vi "Write PID Gains.vi"(0 "VISA Session In":refnum<visa-resource-name>="Alicat", 2 "PID Gain Settings":T1 {"P Gain" min=0 max=65535 step=1; "D Gain" min=0 max=65535 step=1; "I Gain" min=0 max=65535 step=1}, 3 "error in":errorcluster, 4 "Unit ID (A)":string="A") -> (7 "VISA Session Out":refnum<visa-resource-name>, 10 "error out":errorcluster)   [LabVIEW 2016]
doc: "Writes the P, I, and D gains to an Alicat controller."
panel:
  # "Only writes values for \nP, D, & I gains. For other\nvalve tuning options, use \n\"Write PID Settings.vi\""
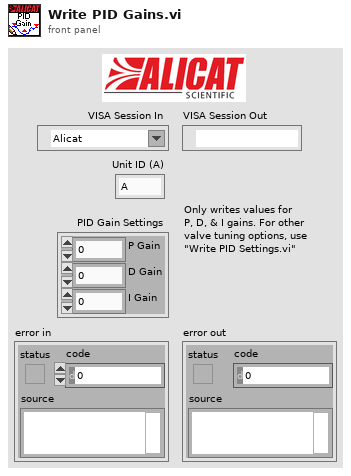
[diagram p1: front panel]
types:
  T1 = cluster{"P Gain":i32, "D Gain":i32, "I Gain":i32}
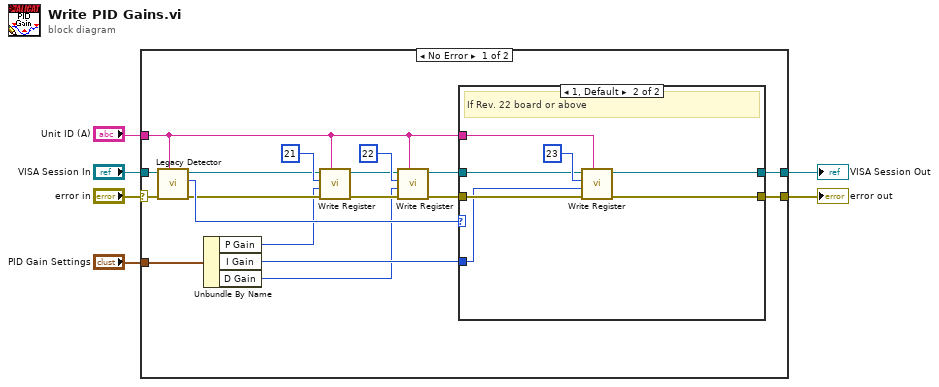
[diagram p0: block diagram]
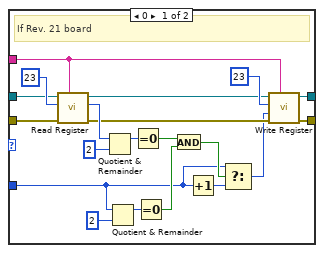
[diagram p2: hidden frame]
diagram:
  n1 = case shown="No Error" "error in" {
    selector: "error in" -> [w23 w52]
    tunnel: [w8 w52] -> w6
    tunnel: [w9 w53] -> w5
    tunnel: "VISA Session In" -> [w24 w53]
    tunnel: "Unit ID (A)" -> [w7 _]
    tunnel: "PID Gain Settings" -> [w22 _]
    frame No Error {
      n2 = call "Legacy Detector.vi"("Unit ID (A)"=w7, "error in"=w23, "VISA Session In"=w24) -> ("error out"=w17:errorcluster, "Legacy Status"=w21:u8, "VISA Session Out"=w16:refnum<visa-resource-name>)  [unwired: 6 in]
      n3 = Unbundle By Name(w22) -> ("P Gain"=w11:i32, "I Gain"=w20:i32, "D Gain"=w10:i32)
      n4 = call "Write Register.vi"("Unit ID (A)"=w7, "error in"=w17, "Register Value"=w11, "Register address"=u16 21, "VISA Session In"=w16) -> ("error out"=w12:errorcluster, "VISA Session Out"=w15:refnum<visa-resource-name>)  [unwired: 4 in, 1 out]
      n5 = call "Write Register.vi"("Unit ID (A)"=w7, "error in"=w12, "Register Value"=w10, "Register address"=u16 22, "VISA Session In"=w15) -> ("error out"=w13:errorcluster, "VISA Session Out"=w14:refnum<visa-resource-name>)  [unwired: 4 in, 1 out]
      n6 = case shown="1, Default" w21 {
        tunnel: w14 -> [w43 w47]
        tunnel: w13 -> [w42 w46]
        tunnel: [w35 w50] -> w8
        tunnel: [w36 w49] -> w9
        tunnel: w7 -> [w33 w48]
        tunnel: w20 -> [w27 w45]
        frame 0 {
          # "If Rev. 21 board"
          n7 = call "Read Register.vi"("Unit ID (A)"=w33, "error in"=w42, "Register address"=u16 23, "VISA Session In"=w43) -> ("error out"=w37:errorcluster, "Register Value (I32)"=w39:i32, "VISA Session Out"=w34:refnum<visa-resource-name>)  [unwired: 5 in]
          n8 = Quotient & Remainder(x=w39, y=2) -> (x-y*floor(x/y)=w40:i32)  [unwired: 1 out]
          n9 = Quotient & Remainder(x=w27, y=2) -> (x-y*floor(x/y)=w31:i32)  [unwired: 1 out]
          n10 = Equal To 0?(x=w40) -> (x = 0?=w30:bool)
          n11 = Equal To 0?(x=w31) -> (x = 0?=w29:bool)
          n12 = And(x=w30, y=w29) -> (x .and. y?=w28:bool)
          n13 = Increment(x=w27) -> (x+1=w26:i32)
          n14 = Select(t=w27, s=w28, f=w26) -> (s? t:f=w25:i32)
          n15 = call "Write Register.vi"("Unit ID (A)"=w33, "error in"=w37, "Register Value"=w25, "Register address"=u16 23, "VISA Session In"=w34) -> ("error out"=w35:errorcluster, "VISA Session Out"=w36:refnum<visa-resource-name>)  [unwired: 4 in, 1 out]
        }
        frame 1, Default {
          # "If Rev. 22 board or above"
          n16 = call "Write Register.vi"("Unit ID (A)"=w48, "error in"=w46, "Register Value"=w45, "Register address"=u16 23, "VISA Session In"=w47) -> ("error out"=w50:errorcluster, "VISA Session Out"=w49:refnum<visa-resource-name>)  [unwired: 4 in, 1 out]
        }
      }
    }
    frame Error {
    }
  }
  "error out" <- w6
  "VISA Session Out" <- w5
